vi "Excel - Append Table Tests.vi"(8 "error in (no error)":errorcluster) -> (0 "error out":errorcluster)   [LabVIEW 2020]
uses:
  src/LabVIEW NPOI/MS-Excel/MS-Excel.lvclass
  D:/Benjamin/Documents/Perso/Code/WC/LabVIEW_NPOI/src/LabVIEW NPOI/Document/Document.lvclass
  src/LabVIEW NPOI/Document/Append Table (string).vi
  src/LabVIEW NPOI/MS-Excel/Get Next Empty Cell.vi
  src/LabVIEW NPOI/Document/Append Table (double).vi
  <vilib>/addons/_JKI Toolkits/Caraya/classes/Assert/Assert Not Error.vi
  <vilib>/addons/_JKI Toolkits/Caraya/classes/Assert/Assert True.vi
  src/LabVIEW NPOI/Document/Document.lvclass
  <vilib>/addons/_JKI Toolkits/Caraya/classes/Test/Test.lvclass
  <vilib>/addons/_JKI Toolkits/Caraya/classes/Assert/Assert.lvclass
  D:/Benjamin/Documents/Perso/Code/WC/LabVIEW_NPOI/src/LabVIEW NPOI/MS-Excel/MS-Excel.lvclass
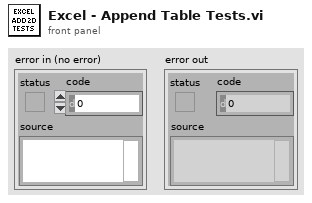
[diagram p1: front panel]
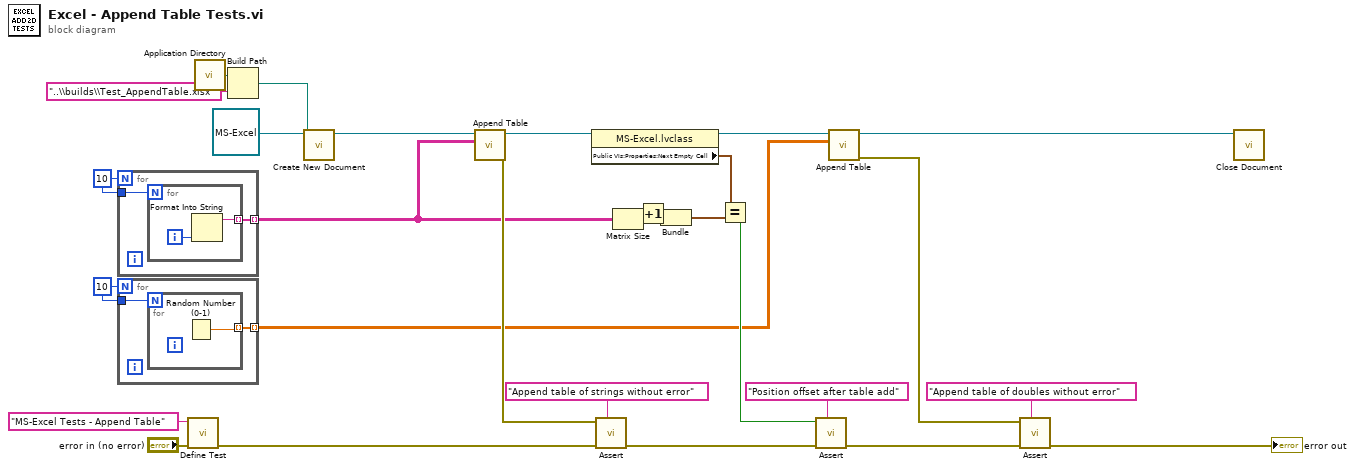
[diagram p0: block diagram]
diagram:
  w6 = 10
  w18 = 10
  n1 = for {
    N: w18 -> [_]
    tunnel: [w31] -> w10 mode=indexing
    tunnel: w18 -> [w30]
    n2 = for {
      N: w30 -> [_]
      tunnel: [w32] -> w31 mode=indexing
      i -> [w33]
      n3 = Format Into String(w33) -> (resulting string=w32:string)  [unwired: 3 in, 1 out]
    }
  }
  n4 = for {
    N: w6 -> [_]
    tunnel: [w35] -> w5 mode=indexing
    tunnel: w6 -> [w34]
    n5 = for {
      N: w34 -> [_]
      tunnel: [w36] -> w35 mode=indexing
      n6 = Random Number (0-1)() -> (number: 0 to 1=w36:dbl)
    }
  }
  n7 = call <vilib>:"Define Test.vi"("error in (no error)"="error in (no error)", "Label (VI Title)"="MS-Excel Tests - Append Table") -> ("error out"=w28:errorcluster)  [unwired: 9 in]
  n8 = call <vilib>:"Application Directory.vi"() -> ("Application Directory"=w22:path)
  n9 = Build Path(base path=w22, name or relative path="..\\builds\\Test_AppendTable.xlsx" ("string")) -> (appended path=w9:path)
  n10 = call "Create New Document.vi"("File Path"=w9, "Document in"=refnum<class "MS-Excel.lvclass"> refnum ("LabVIEW NPOI.lvlib:MS-Excel.lvclass")) -> ("Document out"=w20:refnum<class "MS-Excel.lvclass">)  [unwired: 8 in, 1 out]
  n11 = call-poly "Append Table.vi"("Table"=w10, "Document in"=w20) -> ("error out"=w11:errorcluster, "Document out"=w19:refnum<class "MS-Excel.lvclass">)  [unwired: 8 in]
  n12 = property class="MS-Excel.lvclass"(reference=w19) -> (reference out=w7:refnum<class "MS-Excel.lvclass">, "Public VIs:Properties:Next Empty Cell"=w17:cluster{"Row":i32, "Column":i32})  [unwired: 1 in, 1 out]
  n13 = call-poly <vilib>:"Assert.vi"("Label"="Append table of strings without error", "error in (no error)"=w28, "Not Error?"=w11) -> ("error out"=w26:errorcluster)  [unwired: 8 in]
  n14 = Matrix Size(0:w10) -> (1:w16:i32, 2:w15:i32)
  n15 = Increment(x=w16) -> (x+1=w12:i32)
  n16 = Bundle(w12, "matrix"=w15) -> (w14:cluster{i32, "matrix":i32})  [unwired: 1 in]
  n17 = Equal?(x=w17, y=w14) -> (x = y?=w13:bool)
  n18 = call-poly <vilib>:"Assert.vi"("Label"="Position offset after table add", "error in (no error)"=w26, "True?"=w13) -> ("error out"=w4:errorcluster)  [unwired: 8 in]
  n19 = call-poly "Append Table.vi"("Table"=w5, "Document in"=w7) -> ("error out"=w1:errorcluster, "Document out"=w8:refnum<class "MS-Excel.lvclass">)  [unwired: 8 in]
  n20 = call-poly <vilib>:"Assert.vi"("Label"="Append table of doubles without error", "error in (no error)"=w4, "Not Error?"=w1) -> ("error out"=→"error out":errorcluster)  [unwired: 8 in]
  n21 = call "Close Document.vi"("Document in"=w8) -> ()  [unwired: 10 in, 1 out]
